vi "switchmodetest.vi"() -> ()   [LabVIEW 2015]
uses:
  BERTTA.dll
panel:
  in  "Boolean":bool
  in  "mode":i32
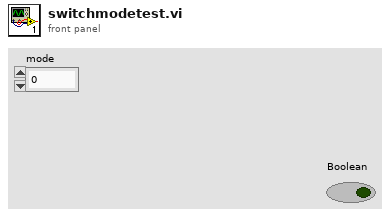
[diagram p1: front panel]
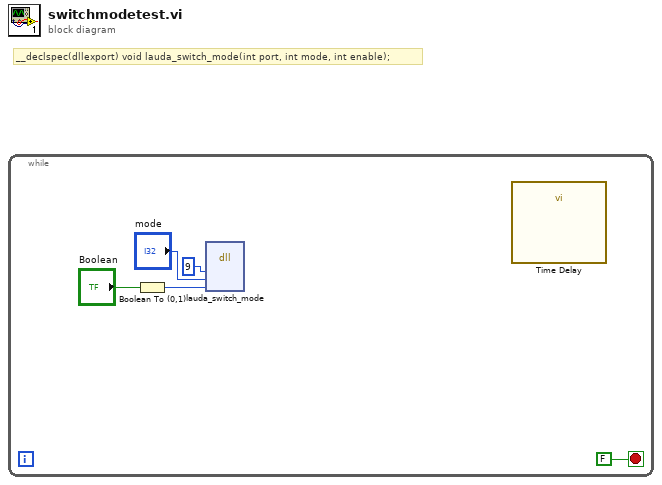
[diagram p0: block diagram]
diagram:
  # "__declspec(dllexport) void lauda_switch_mode(int port, int mode, int enable);"
  n1 = while {
    stop <- FALSE stop-if-true
    n2 = Boolean To (0,1)(Boolean="Boolean") -> (0, 1=w2:i16)
    n3 = dll-call lib="C:/Users/shresplab/OneDrive - Kemira Oyj/Documents/Visual Studio 2017/Projects/Bertta/BERTTA/x64/Debug/BERTTA.dll" fn="lauda_switch_mode"("port"=9, "mode"="mode", "enable"=w2) -> ()  [unwired: 7 in, 2 out]
    n4 = call "Time Delay"() -> ()  [unwired: 11 in, 1 out]
  }
